vi "Image or Table Caption.vi"(0 "PDF Report IN":refnum<class "PDF Report Class.lvclass">, 2 "Image or Table":T1, 9 "Caption IN":string, 11 "error IN":errorcluster) -> (4 "PDF Report OUT":refnum<class "PDF Report Class.lvclass">, 6 "Paragraph Refnum":refnum<k24>, 15 "error OUT":errorcluster)   [LabVIEW 2019, in "Exaprom PDF.lvlib"]
doc: "Version 2.0\nDeveloped by Jean-Marc Simard\nCopyright © 2012, Exaprom Inc.\nAll rights reserved.\nLicense: BSD\n\nWith iTextSharp 4.1.6 (http://itextsharp.sourceforge.net)\nunder Mozilla Public License Version 1.1\n(http://www.mozilla.org/MPL/MPL-1.1.html)"
uses:
  LV Class/PDF Report Class/PDF Report Class.lvclass
  C:/work/niobrara_lv/labview pdf writer fixing/DLL/itextsharp.dll
  DLL/itextsharp.dll
  Not  in the library/Images for controls/Image or Table.ctl
  Controls/Initialization Controls/Defaut Paragraphe and Line Spacing.ctl
  Controls/Text Controls/Line spacing.ctl
  Exaprom PDF.lvlib
  LV Class/Fonts Class/Font Class.lvclass
  Controls/Text Controls/Texte alignement.ctl
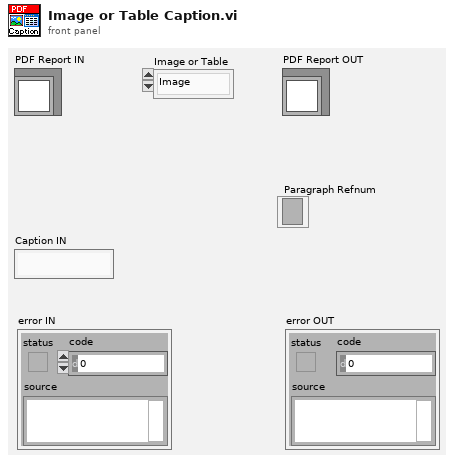
[diagram p1: front panel]
types:
  T1 = typedef "Exaprom PDF.lvlib/Image or Table.ctl" = enum16{"Image", "Table"}
  T2 = typedef "Exaprom PDF.lvlib/Defaut Paragraphe and Line Spacing.ctl" = cluster{" Aligment":T3, "Line spacing":T4}
  T3 = typedef "Exaprom PDF.lvlib/Texte alignement.ctl" = enum16{"Select", "CENTER", "JUSTIFY", "LEFT", "RIGHT"}
  T4 = typedef "Exaprom PDF.lvlib/Line spacing.ctl" = enum16{"Select", "1.0", "1.5", "2.0"}
  T5 = typedef "Exaprom PDF.lvlib/Font complete cluster.ctl" = cluster{"Name":string, "Size":T6, "Color":T7, "Style":cluster{"Bold":bool, "Italic":bool, "Underline":bool, "Strikeout":bool}, "Type":T8}
  T6 = typedef "Exaprom PDF.lvlib/Font size.ctl" = sgl
  T7 = typedef "Exaprom PDF.lvlib/Font color.ctl" = u32
  T8 = typedef "Exaprom PDF.lvlib/Type and encoding.ctl" = cluster{"Type&direction":T9, "Embedded":bool, "Encoding":string}
  T9 = typedef "Exaprom PDF.lvlib/Type and run direction.ctl" = enum16{"Select", "ASCII", "UTF-16", "UTF-16 (default)", "UTF-16 (LTR)", "UTF-16 (RTL)"}
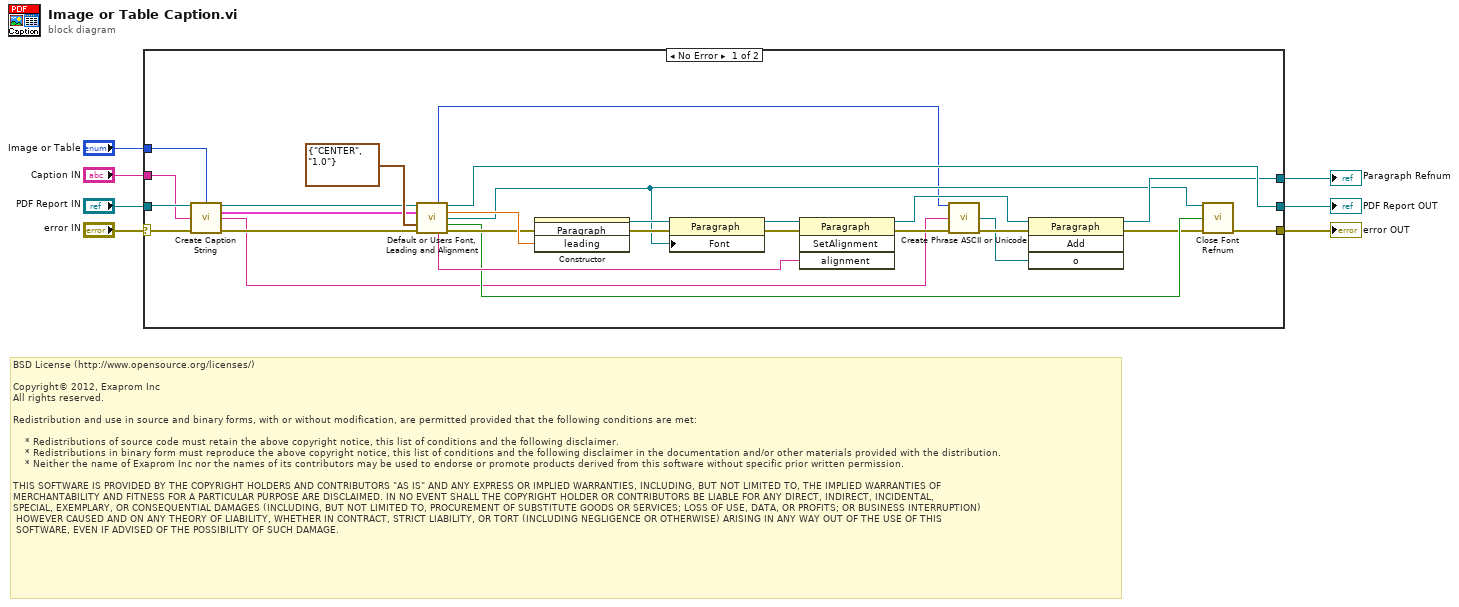
[diagram p0: block diagram]
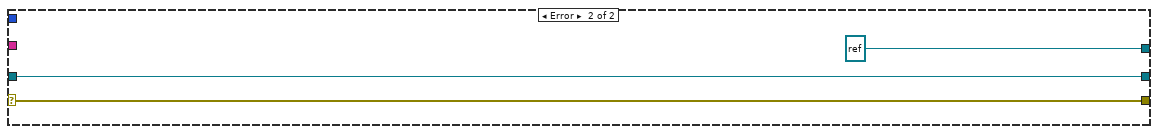
[diagram p2: hidden frame]
diagram:
  # "BSD License (http://www.opensource.org/licenses/)\n\nCopyright© 2012, Exaprom Inc\nAll rights reserved.\n\nRedistribution and use in source and binary forms, with or without modification, are permitted provided that the following conditions are met:\n\n    * Redistributions of source code must retain the above copyright notice, this list of conditions and the following disclaimer.\n    * Redistributions in binary form must reproduce the above copyright notice, this list of conditions and the following disclaimer in the documentation and/or other materials provided with the distribution.\n    * Neither the name of Exaprom Inc nor the names of its contributors may be used to endorse or promote products derived from this software without specific prior written permission.\n\nTHIS SOFTWARE IS PROVIDED BY THE COPYRIGHT HOLDERS AND CONTRIBUTORS \"AS IS\" AND ANY EXPRESS OR IMPLIED WARRANTIES, INCLUDING, BUT NOT LIMITED TO, THE IMPLIED WARRANTIES OF \nMERCHANTABILITY AND FITNESS FOR A PARTICULAR PURPOSE ARE DISCLAIMED. IN NO EVENT SHALL THE COPYRIGHT HOLDER OR CONTRIBUTORS BE LIABLE FOR ANY DIRECT, INDIRECT, INCIDENTAL,\nSPECIAL, EXEMPLARY, OR CONSEQUENTIAL DAMAGES (INCLUDING, BUT NOT LIMITED TO, PROCUREMENT OF SUBSTITUTE GOODS OR SERVICES; LOSS OF USE, DATA, OR PROFITS; OR BUSINESS INTERRUPTION)\n HOWEVER CAUSED AND ON ANY THEORY OF LIABILITY, WHETHER IN CONTRACT, STRICT LIABILITY, OR TORT (INCLUDING NEGLIGENCE OR OTHERWISE) ARISING IN ANY WAY OUT OF THE USE OF THIS\n SOFTWARE, EVEN IF ADVISED OF THE POSSIBILITY OF SUCH DAMAGE."
  n1 = case shown="No Error" "error IN" {
    selector: "error IN" -> [w25 w37]
    tunnel: [w26 w36] -> w7
    tunnel: "Caption IN" -> [w23 _]
    tunnel: "PDF Report IN" -> [w24 w36]
    tunnel: [w27 w37] -> w4
    tunnel: [w17 refnum<k24> refnum ("new reference")] -> w2
    tunnel: "Image or Table" -> [w10 _]
    frame No Error {
      n2 = call "Create Caption String.vi"("PDF Report IN"=w24, "Image or Table"=w10, "Caption IN"=w23, "error in (no error)"=w25) -> ("PDF Report OUT"=w29:refnum<class "PDF Report Class.lvclass">, "Font"=w9:T5, "Caption OUT"=w15:string, "error out"=w28:errorcluster)  [unwired: 8 in]
      n3 = call "Default or Users Font, Leading and Alignment.vi"("PDF Report"=w29, "Font"=w9, "Paragraphe cluster"=T2 {" Aligment"=enum."CENTER", "Line spacing"=enum."1.0"}, "error in (no error)"=w28) -> ("Type and run direction"=w8:T9, "PDF Report duplicate"=w26:refnum<class "PDF Report Class.lvclass">, "Leading"=w33:T6, "Font Ref"=w12:refnum<k24>, "Close Font Ref"=w30:bool, "Aligment"=w31:string, "error out"=w32:errorcluster)  [unwired: 5 out]
      n4 = constructor class="Paragraph"(error in=w32, "leading"=w33) -> (reference out=w21:refnum<k24>, error out=w22:errorcluster)  [unwired: 2 in, 2 out]
      n5 = property class="Paragraph"(reference=w21, error in=w22, "Font"=w12) -> (reference out=w19:refnum<k24>, error out=w20:errorcluster)
      n6 = invoke class="Paragraph" method="SetAlignment"(reference=w19, error in=w20, "alignment"=w31) -> (reference out=w11:refnum<k24>, error out=w16:errorcluster)  [unwired: 1 in, 2 out]
      n7 = call "Create Phrase ASCII or Unicode.vi"("Character type"=w8, "Text"=w15, "error in (no error)"=w16) -> ("Phrase refnum"=w13:refnum<k24>, "error out"=w14:errorcluster)  [unwired: 10 in, 1 out]
      n8 = invoke class="Paragraph" method="Add"(reference=w11, error in=w14, "o"=w13) -> (reference out=w17:refnum<k24>, error out=w18:errorcluster)  [unwired: 1 in, 2 out]
      n9 = call "Close Font Refnum.vi"("Font Refnum"=w12, "Close ?"=w30, "error in (no error)"=w18) -> ("error out"=w27:errorcluster)  [unwired: 12 in]
    }
    frame Error {
    }
  }
  "PDF Report OUT" <- w7
  "error OUT" <- w4
  "Paragraph Refnum" <- w2
